vi "add set gating(SubVI).vi"(10 "字符串":string) -> (1 "ok or cancel":bool=TRUE, 2 "连接的字符串":string)   [LabVIEW 2019, in "SubVI.lvlib"]
uses:
  SubVI.lvlib
panel:
  in  "Amplitude":dbl
  in  "cancel":bool
  in  "ok":bool
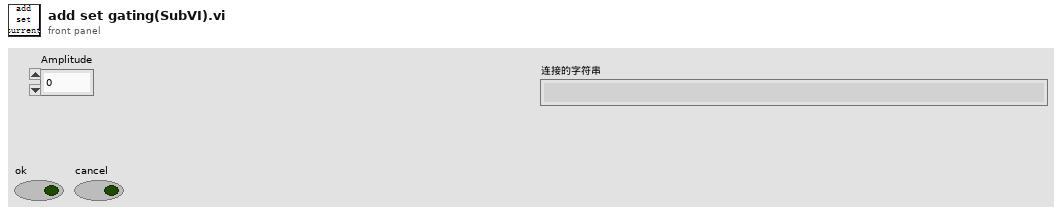
[diagram p1: front panel]
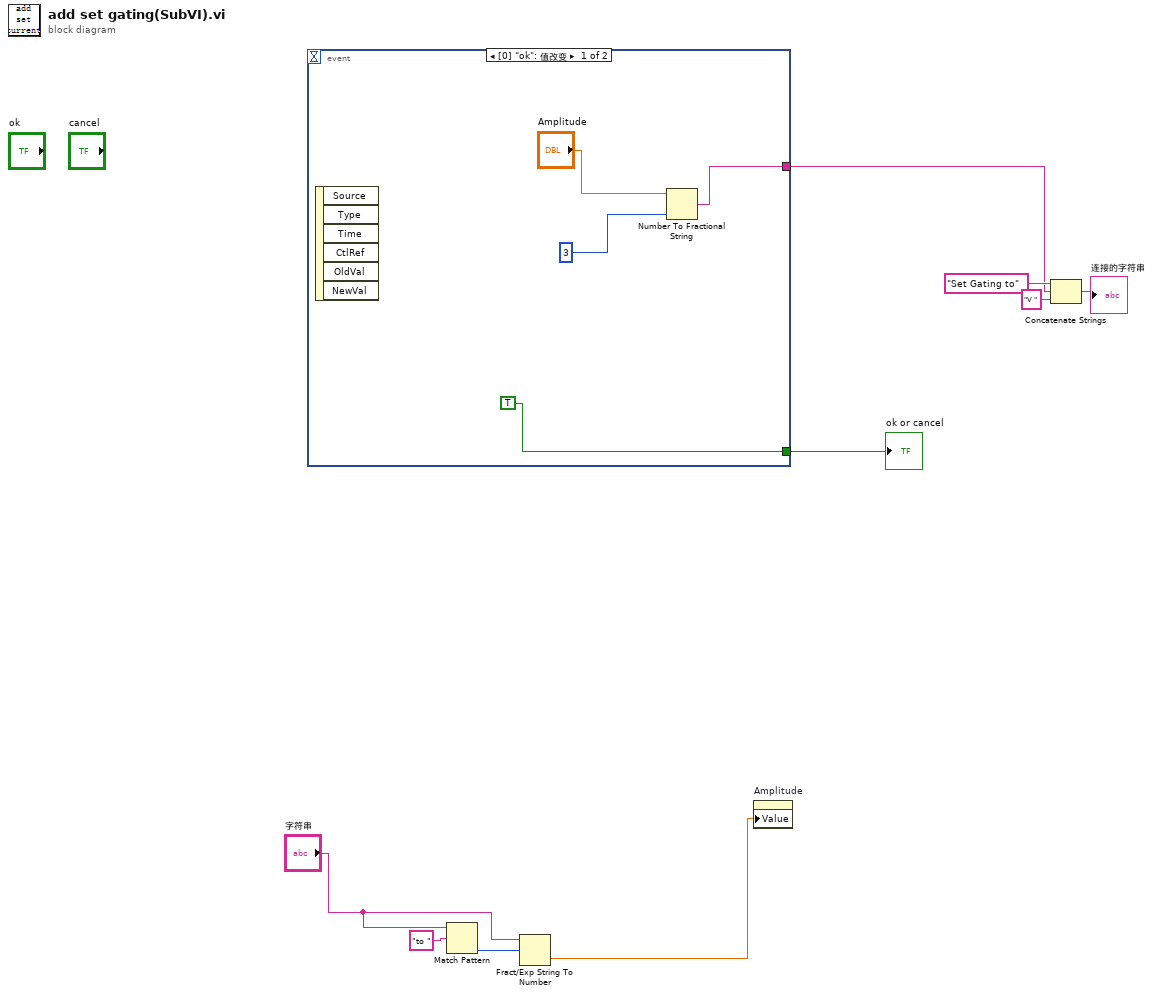
[diagram p0: block diagram]
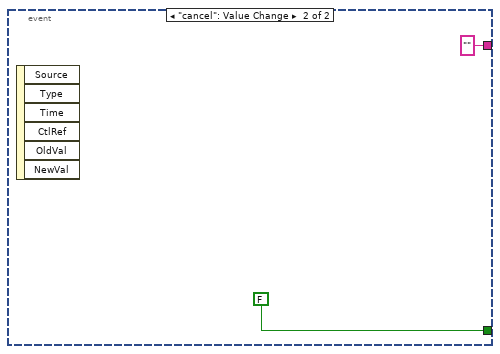
[diagram p2: hidden frame]
diagram:
  n1 = event shown="[0] \"ok\": 值改变" {
    selector: _ -> [_ _]
    dyn-events: _ -> [_ _]
    timeout: _ -> [_ _]
    tunnel: [TRUE FALSE] -> w7
    tunnel: [w10 ""] -> w5
    event "ok": Value Change {
      n2 = event-data() -> ()  [unwired: 1 in, 6 out]
      n3 = Number To Fractional String(number="Amplitude", precision (6)=i16 3 ("精度(6)")) -> (F-format string=w10:string)  [unwired: 2 in]
    }
    event "cancel": Value Change {
      n4 = event-data() -> ()  [unwired: 1 in, 6 out]
    }
  }
  "ok or cancel" <- w7
  n5 = Match Pattern(string="字符串", regular expression="to " ("正则表达式")) -> (offset past match=w3:i32)  [unwired: 1 in, 3 out]
  n6 = Fract/Exp String To Number(string="字符串", offset=w3) -> (number=w1:dbl)  [unwired: 2 in, 1 out]
  n7 = property on="Amplitude" class="DigNum (严格)"("Value"=w1) -> ()  [unwired: 2 in, 2 out]
  n8 = Concatenate Strings("Set Gating to" ("字符串"), w5, "V " ("字符串")) -> (→"连接的字符串":string)
